vi "update log.vi"(11 "更新记录":string) -> (3 "check":bool)   [LabVIEW 2016, in "数据传输系统-03.lvlib" / "update.lvlib"]
uses:
  update.lvlib
panel:
  out "计时":i32
  in  "取消":bool
  in  "布尔":bool
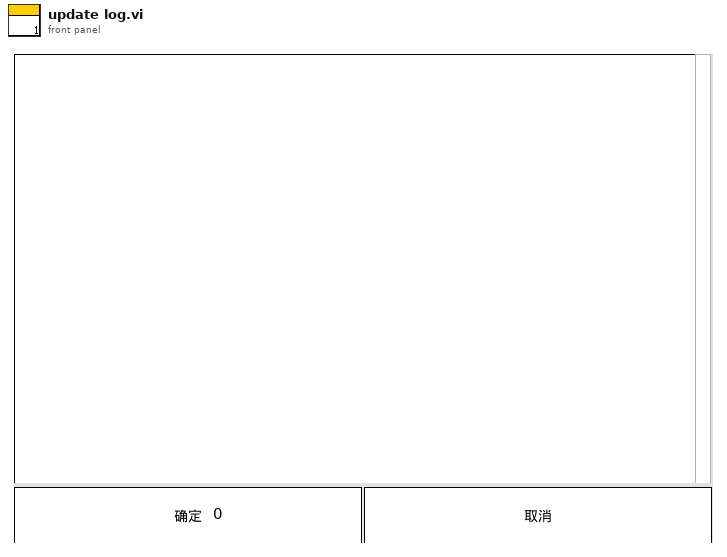
[diagram p1: front panel]
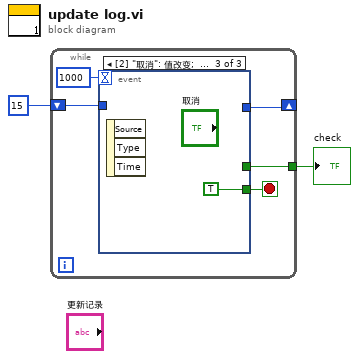
[diagram p0: block diagram]
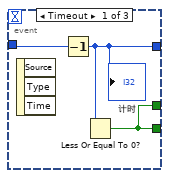
[diagram p2: hidden frame]
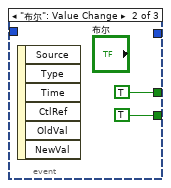
[diagram p3: hidden frame]
diagram:
  n1 = while {
    tunnel: [w6] -> w2
    shift-right: [w4] -> _
    shift-left: 15 -> [w5]
    stop <- w7 stop-if-true
    n2 = event shown="[2] \"取消\": 值改变;  前面板关闭" {
      selector: _ -> [_ _ _]
      dyn-events: _ -> [_ _ _]
      timeout: 1000 -> [_ _ _]
      tunnel: [w8 TRUE TRUE] -> w7
      tunnel: [w8 TRUE _] -> w6
      tunnel: w5 -> [w10 _ _]
      tunnel: [w9 _ _] -> w4
      event Timeout {
        n3 = event-data() -> ()  [unwired: 1 in, 3 out]
        n4 = Decrement(x=w10) -> (x-1=w9:i32)
        "计时" <- w9
        n5 = Less Or Equal To 0?(x=w9) -> (x <= 0?=w8:bool)
      }
      event "布尔": Value Change {
        n6 = event-data() -> ()  [unwired: 1 in, 6 out]
      }
      event "取消": Value Change; Panel Close {
        n7 = event-data() -> ()  [unwired: 1 in, 3 out]
      }
    }
  }
  "check" <- w2
